vi "GFITS_LibHeaders.vi"(6 "memheaders":bool, 7 "file ref":u64, 8 "error in (no error)":errorcluster, 9 "funtion name":string, 10 "Table In":string[][](table), 11 "data type":i32[](array[numeric])) -> (0 "error out":errorcluster)   [LabVIEW 2016]
uses:
  c/lib/libgfits.so
panel:
  out "output param 2":i32
  out "output param":i32
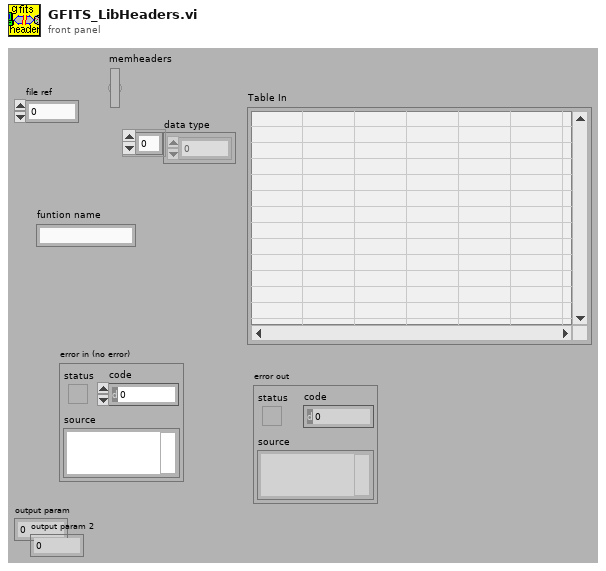
[diagram p1: front panel]
types:
  T1 = enum16{"clear all", "add extension", "add keyword", "get", "clear extension", "done"}
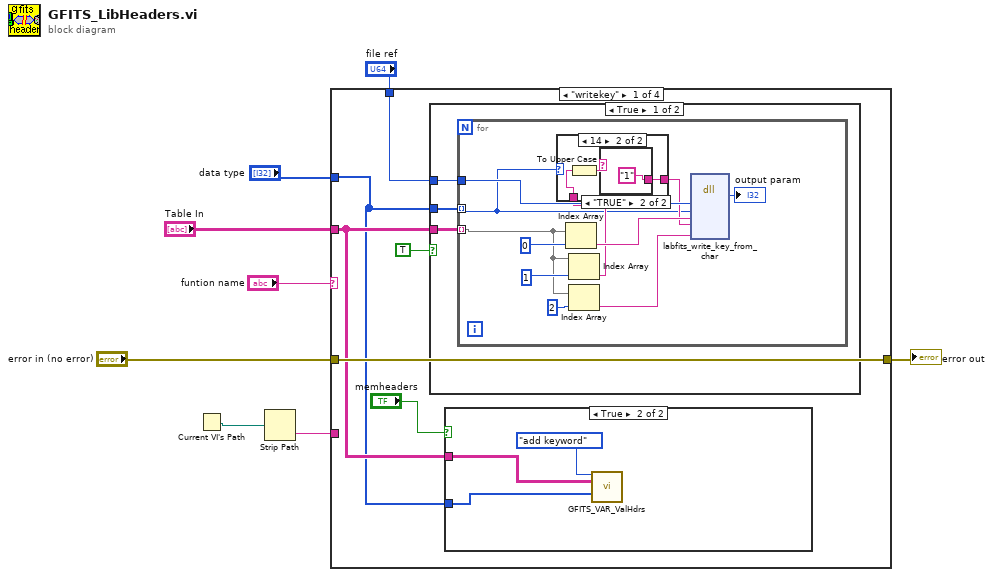
[diagram p0: block diagram]
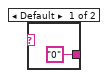
[diagram p4: hidden frame]
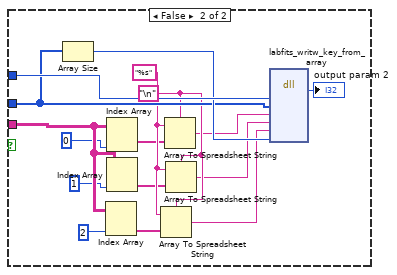
[diagram p5: hidden frame]
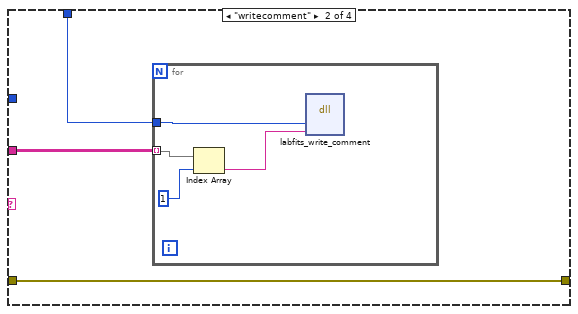
[diagram p6: hidden frame]
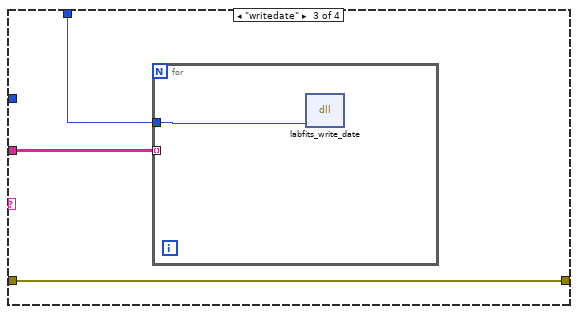
[diagram p7: hidden frame]
diagram:
  n1 = Current VI's Path() -> (path=w1:path)
  n2 = Strip Path(path=w1) -> (name=w2:string)  [unwired: 1 out]
  n3 = case shown="\"writekey\"" "funtion name" {
    tunnel: "file ref" -> [w13 w56 w63 _]
    tunnel: "data type" -> [w9 _ _ _]
    tunnel: "Table In" -> [w10 w55 w62 _]
    tunnel: "error in (no error)" -> [w14 w54 w61 w65]
    tunnel: [w14 w54 w61 w65] -> w4
    tunnel: w2 -> [_ _ _ _]
    frame "writekey" {
      n4 = case shown="True" TRUE {
        tunnel: w10 -> [w20 w53]
        tunnel: w9 -> [w19 w46]
        tunnel: w13 -> [w18 w52]
        frame True {
          n5 = for {
            tunnel: w19 -> [w21] mode=indexing
            tunnel: w20 -> [w27] mode=indexing
            tunnel: w18 -> [w24]
            n6 = Index Array(array=w27, index=0) -> (element=w26:string)
            n7 = Index Array(array=w27, index=1) -> (element=w23:string)
            n8 = case shown="14" w21 {
              tunnel: w23 -> [w32 w35]
              tunnel: [w32 w33] -> w22
              frame Default {
              }
              frame 14 {
                n9 = To Upper Case(1:w35) -> (0:w34:string)
                n10 = case shown="\"TRUE\"" w34 {
                  tunnel: ["0" "1"] -> w33
                  frame Default {
                  }
                  frame "TRUE" {
                  }
                }
              }
            }
            n11 = Index Array(array=w27, index=2) -> (element=w25:string)
            n12 = dll-call lib="home/simager/panview/PAN/Modules/GFITS/private/c/lib/libgfits.so" fn="labfits_write_key_from_char"("ref"=w24, "datatype"=w21, "keyname"=w26, "value"=w22, "comment"=w25) -> ("return type"=→"output param":i32)  [unwired: 8 in, 2 out]
          }
        }
        frame False {
          w44 = "\n" ("delimiter (Tab)")
          w45 = "%s" ("format string")
          n13 = Array Size(array=w46) -> (size(s)=w47:i32)
          n14 = Index Array(array=w53, index (col)=2) -> (element=w41:string[])  [unwired: 1 in]
          n15 = Index Array(array=w53, index (col)=0) -> (element=w43:string[])  [unwired: 1 in]
          n16 = Index Array(array=w53, index (col)=1) -> (element=w42:string[])  [unwired: 1 in]
          n17 = Array To Spreadsheet String(delimiter (Tab)=w44, array=w41, 3:w45) -> (spreadsheet string=w38:string)
          n18 = Array To Spreadsheet String(delimiter (Tab)=w44, array=w43, 3:w45) -> (spreadsheet string=w40:string)
          n19 = Array To Spreadsheet String(delimiter (Tab)=w44, array=w42, 3:w45) -> (spreadsheet string=w39:string)
          n20 = dll-call lib="home/simager/panview/PAN/Modules/GFITS/private/c/lib/libgfits.so" fn="labfits_writw_key_from_array"("ref"=w52, "datatype"=w46, "keyname"=w40, "value"=w39, "comment"=w38, "nkeys"=w47) -> ("return type"=→"output param 2":i32)  [unwired: 9 in, 2 out]
        }
      }
      n21 = case shown="True" "memheaders" {
        tunnel: w10 -> [_ w17]
        tunnel: w9 -> [_ w16]
        frame False {
        }
        frame True {
          n22 = call "GFITS_VAR_ValHdrs.vi"("action"=T1."add keyword", "header in"=w17, "data type"=w16) -> ()  [unwired: 2 in, 11 out]
        }
      }
    }
    frame "writecomment" {
      n23 = for {
        tunnel: w56 -> [w60]
        tunnel: w55 -> [w59] mode=indexing
        n24 = Index Array(array=w59, index=1) -> (element=w57:string)
        n25 = dll-call lib="home/simager/panview/PAN/Modules/GFITS/private/c/lib/libgfits.so" fn="labfits_write_comment"("ref"=w60, "comment"=w57) -> ()  [unwired: 4 in, 4 out]
      }
    }
    frame "writedate" {
      n26 = for {
        tunnel: w63 -> [w64]
        tunnel: w62 -> [_] mode=indexing
        n27 = dll-call lib="home/simager/panview/PAN/Modules/GFITS/private/c/lib/libgfits.so" fn="labfits_write_date"("ref"=w64) -> ()  [unwired: 4 in, 3 out]
      }
    }
    frame Default {
    }
  }
  "error out" <- w4
